vi "main_host.vi"() -> ()   [LabVIEW 2020]
uses:
  Status Cluster STYP.ctl
  Snake/Snake.lvclass
  INIFile/INIScoreFile.lvclass
  Drawing Settings STYP.ctl
  Food/Food.lvclass
  <userlib>/JET Engineering/JET_QSM/Code/Private/JET_QSM_InvalidOption STYP.ctl
  Direction STYP.ctl
  <userlib>/JET Engineering/JET_QSM/Code/Private/JET_QSM - Add State [String API].vi
  <vilib>/numeric/Random Number (Range) U64.vi
  <vilib>/numeric/sub_Random U32.vi
  <vilib>/Utility/error.llb/Trim Whitespace.vi
  <vilib>/Utility/error.llb/Error Cluster From Error Code.vi
panel:
  out "HighScores":i32(listbox)
  out "Score":u32
  out "Recent states before Error (with tick counts) 2":string="0.167 sec ago: VI Initialize\n0.167 sec ago: Window Open\n0.110 sec ago: Control Update\n0.110 sec ago: Indicator Update\n0.000 sec ago: Error Handler\r\n"
  in  "Status":T1
  out "error out":errorcluster
  out "Play Area":picture
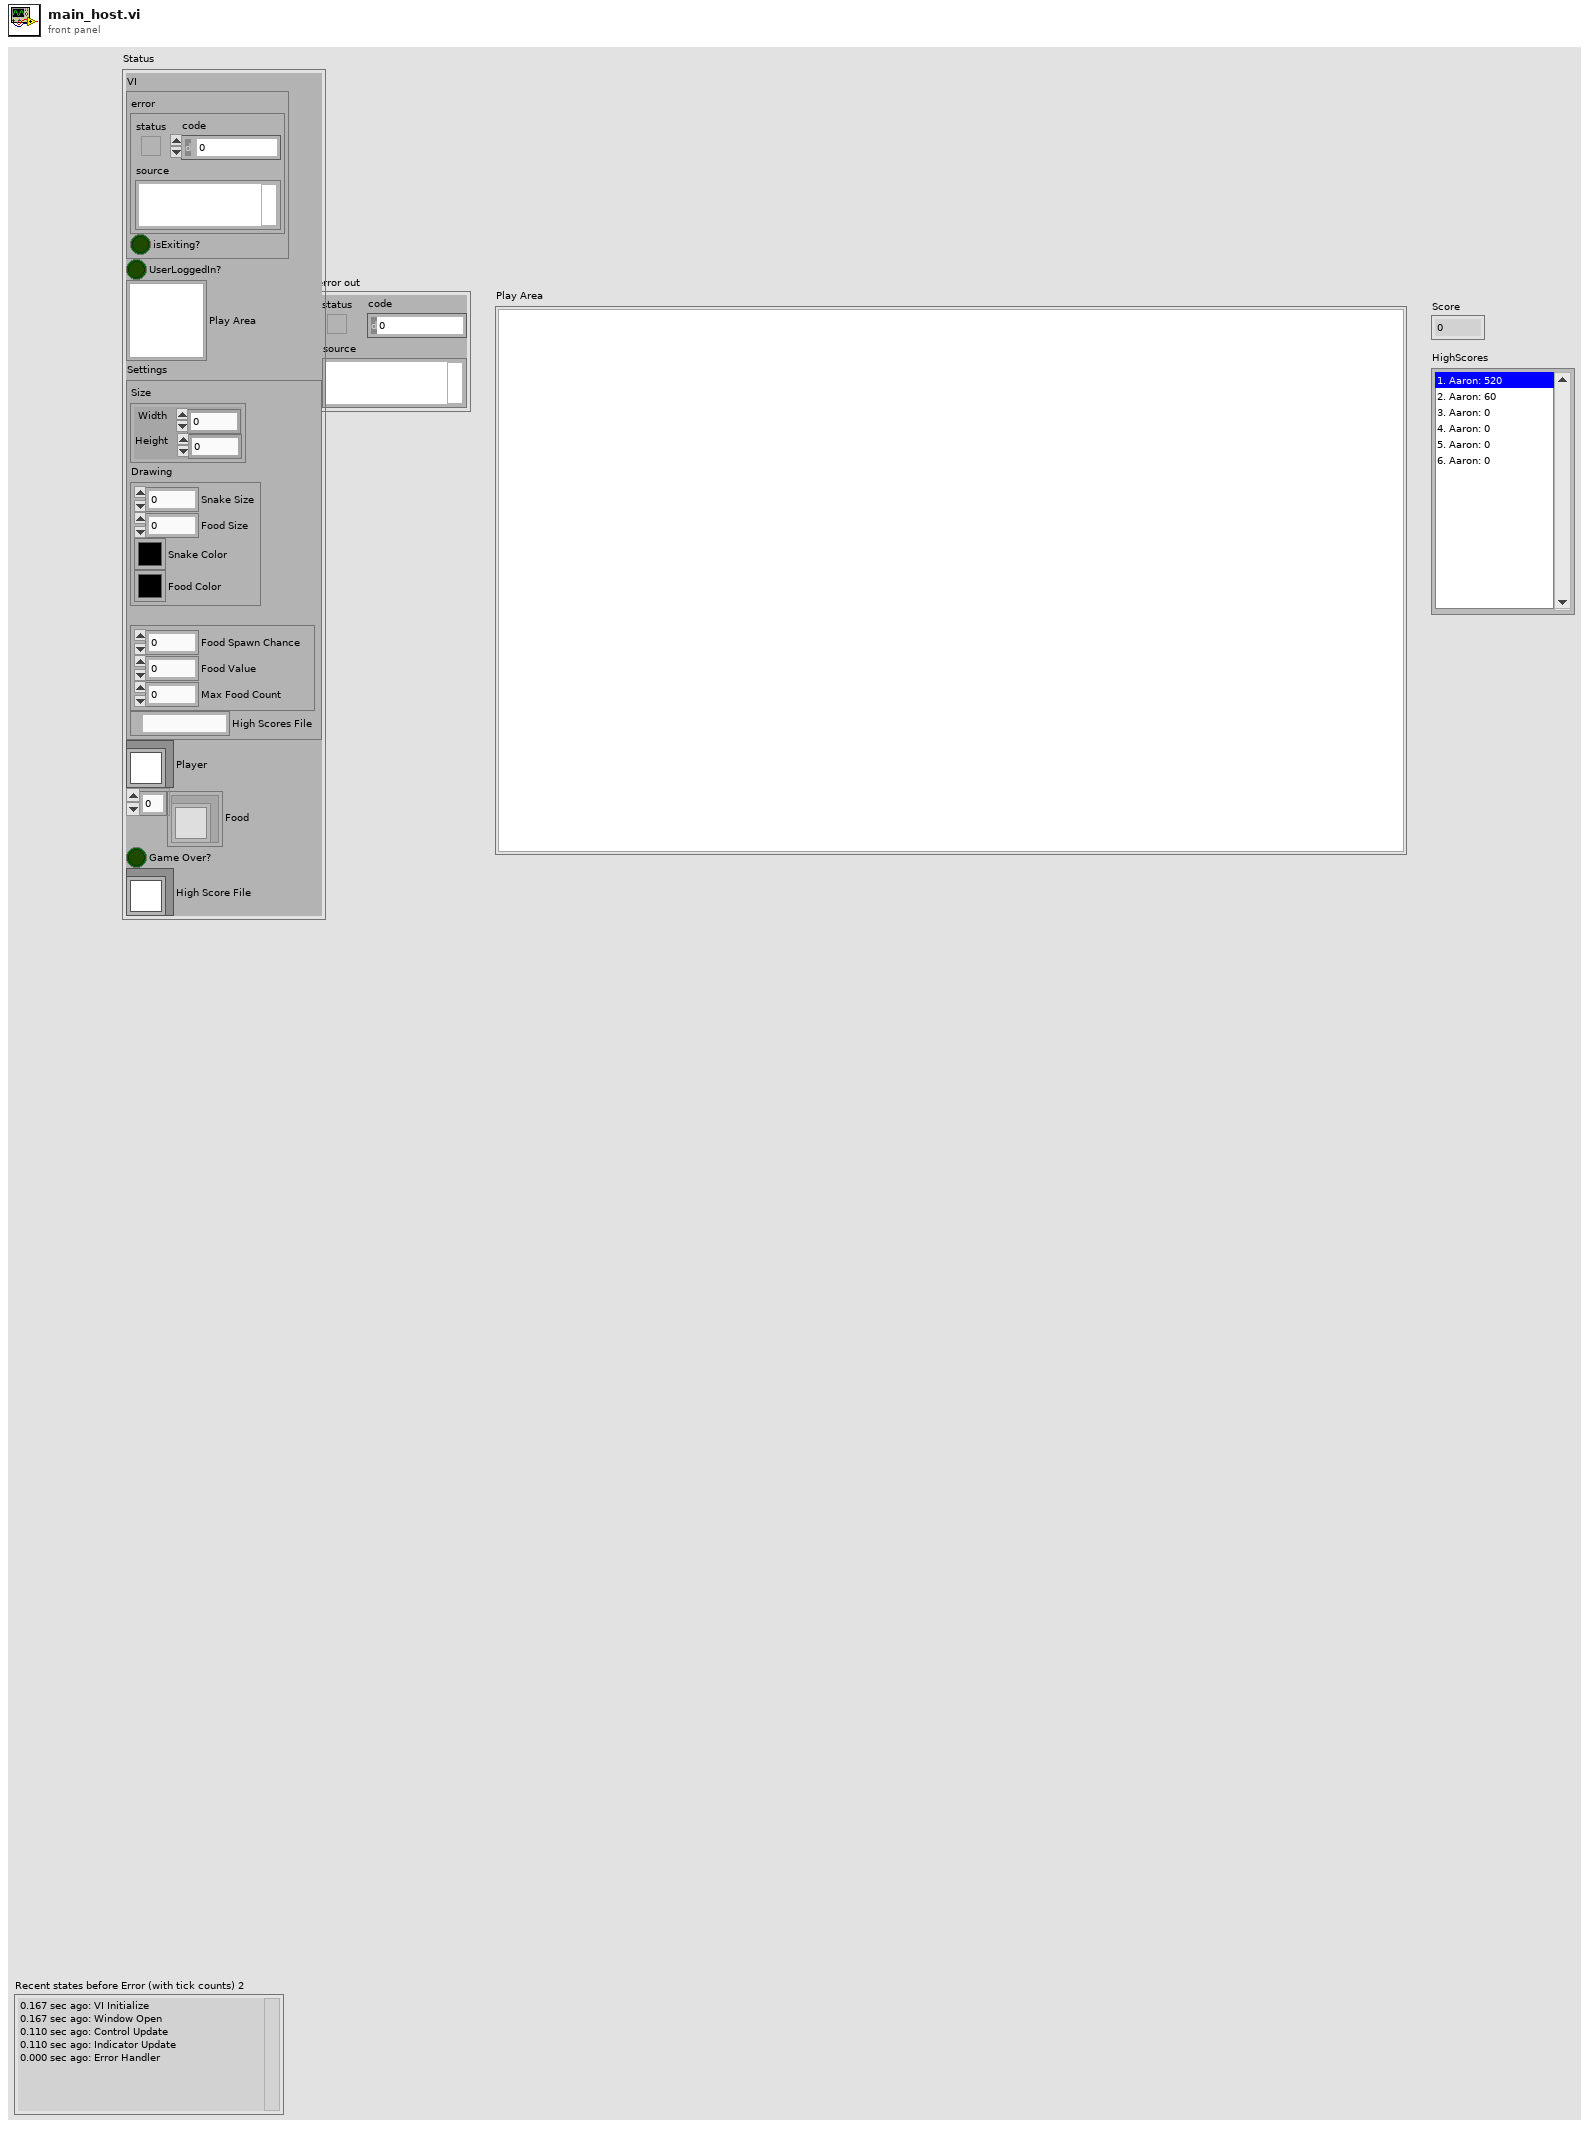
[diagram p1: front panel]
types:
  T1 = typedef "Status Cluster STYP.ctl" = cluster{"VI":cluster{"error":errorcluster, "isExiting?":bool}, "UserLoggedIn?":bool, "Play Area":picture, "Settings":cluster{"Size":cluster{"Width":u32, "Height":u32}, "Drawing":T2, "Food":cluster{"Food Spawn Chance":dbl, "Food Value":u32, "Max Food Count":i32}, "High Scores File":path}, "Player":refnum<class "Snake.lvclass">, "Food":refnum<class "Food.lvclass">[], "Game Over?":bool, "High Score File":refnum<class "INIScoreFile.lvclass">}
  T2 = typedef "Drawing Settings STYP.ctl" = cluster{"Snake Size":u32, "Food Size":u32, "Snake Color":u32, "Food Color":u32}
  T3 = typedef "JET_QSM_InvalidOption STYP.ctl" = enum16{"Ignore", "Dialog", "Error"}
  T4 = typedef "JET_QSM_Refnum STYP.ctl" = cluster{"state":cluster{"queue":refnum<queue>, "idle":string, "error":string, "STOP":string}, "debug":cluster{"enabled?":bool, "queue":refnum<queue>}, "Invalid.option":T3, "QSM.Name":string}
  T5 = enum32{"invalid app kind", "Development System", "Run Time System", "Student Edition", "Embedded LabVIEW", "Evaluation", "Custom"}
  T6 = typedef "Direction STYP.ctl" = enum16{"Up", "Down", "Left", "Right"}
  T7 = typedef "LVBoundsTypeDef.ctl" = cluster{"Width":u32, "Height":u32}
  T8 = typedef "eventvkey.ctl" = enum16{"ASCII", "Enter", "Return", "Shift", "Ctrl", "Alt", "Cmd", "Opt", "Caps", "NumLock", "Clear", "Break", "Up", "Down", "Left", "Right", "Insert", "Delete", "Home", "End", "PageUp", "PageDown", "Escape", "Help", "Pause", "ScrollLock", "F1", "F2", "F3", "F4", "F5", "F6", "F7", "F8", "F9", "F10", "F11", "F12", "F13", "F14", "F15", "F16", "F17", "F18", "F19", "F20", "F21", "F22", "F23", "F24", "Play", "VolumeUp", "VolumeDown", "Mute", "Two Byte Char"}
  T9 = typedef "JET_QSM_Element STYP.ctl" = cluster{"state":string, "data":variant, "comment":string}
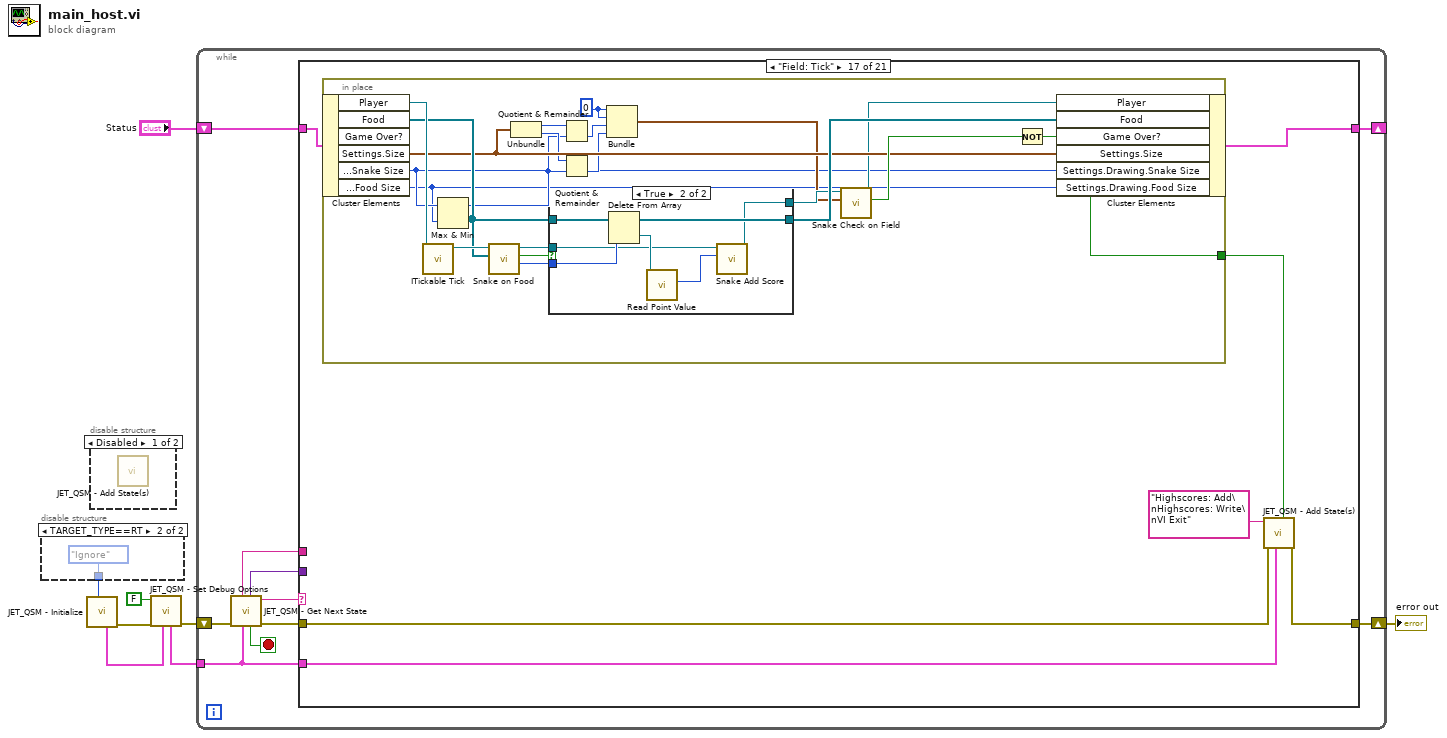
[diagram p0: block diagram]
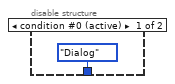
[diagram p2: hidden frame]
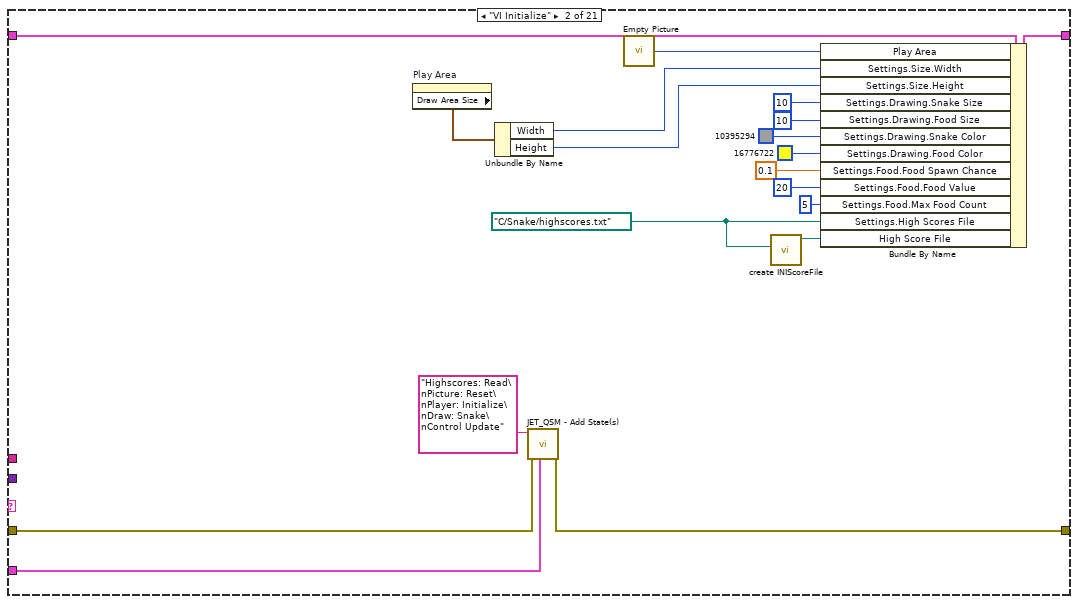
[diagram p5: hidden frame]
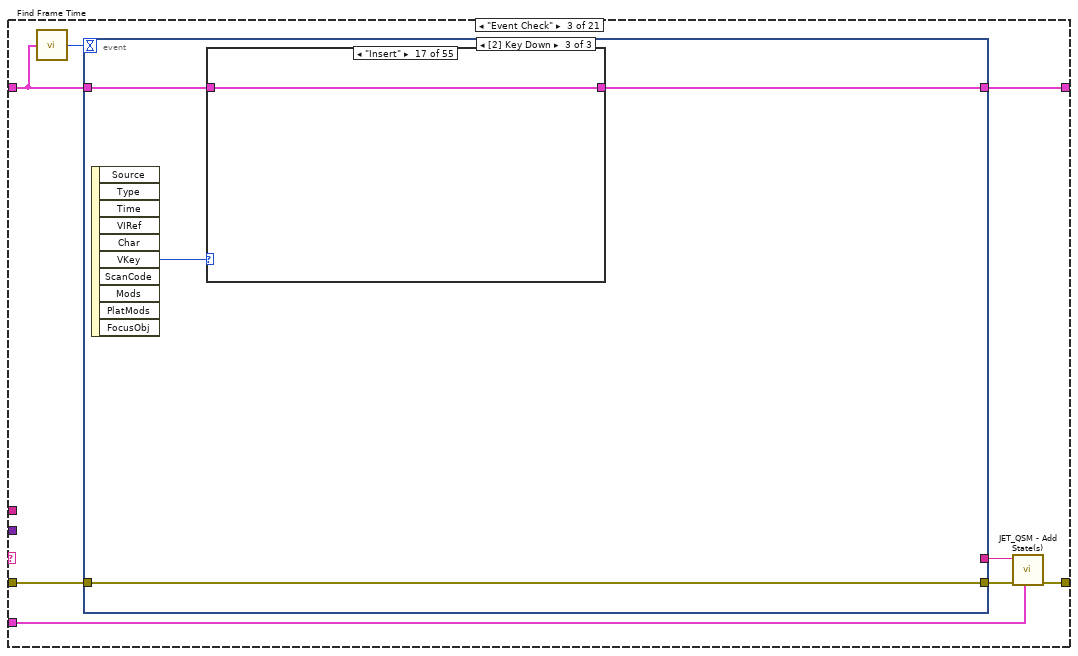
[diagram p6: hidden frame]
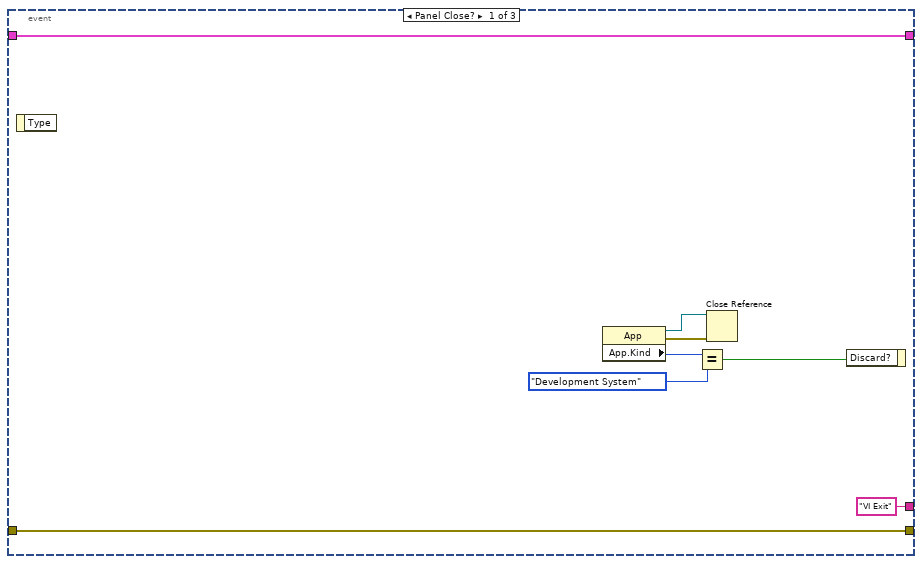
[diagram p7: hidden frame]
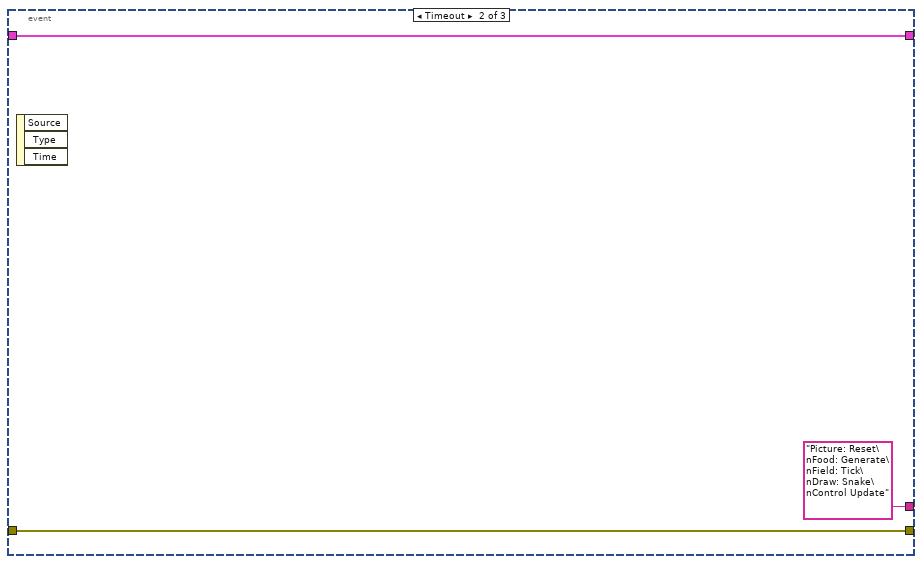
[diagram p8: hidden frame]
diagram:
  n1 = disable-structure shown="TARGET_TYPE==RT" {
    disable-tunnel: [JET_QSM_InvalidOption_STYP."Dialog" ("invalid state action (Dialog)") JET_QSM_InvalidOption_STYP."Ignore" ("invalid state action (Dialog)")] -> w8
    frame condition #0 (active) {
    }
    frame condition #1 {
    }
  }
  n2 = call <userlib>:"JET_QSM - Initialize.vi"("invalid state action (Dialog)"=w8) -> ("error out"=w1:errorcluster, "Jet_QSM refnum"=w4:T4)  [unwired: 9 in]
  n3 = disable-structure shown="Disabled" {
    frame Disabled {
      n4 = call-poly <userlib>:"JET_QSM - Add State(s).vi"() -> ()  [unwired: 11 in, 1 out]
    }
    frame Enabled {
    }
  }
  n5 = call <userlib>:"JET_QSM - Set Debug Options.vi"("Jet_QSM refnum"=w4, "error in (no error)"=w1, "debug.enabled? (F)"=FALSE) -> ("error out"=w2:errorcluster, "Jet_QSM ref"=w3:T4)  [unwired: 7 in]
  n6 = while {
    tunnel: w3 -> [w16]
    shift-right: [w14] -> _
    shift-left: "Status" -> [w15]
    shift-right: [w13] -> w7
    shift-left: w2 -> [w20]
    stop <- w17 stop-if-true
    n7 = call <userlib>:"JET_QSM - Get Next State.vi"("Jet_QSM refnum"=w16, "error in (no error)"=w20) -> ("error out"=w19:errorcluster, "state"=w18:string, "Stop Loop?"=w17:bool, "state data"=w12:variant, "state comment"=w11:string)  [unwired: 5 in]
    n8 = case shown="\"Field: Tick\"" w18 {
      selector: w18 -> [_ _ _ _ _ _ w176 _ _ _ _ _ _ _ _ _ _ _ _ _ _]
      tunnel: w19 -> [w21 w35 w49 w137 w168 _ w177 w179 w181 w183 w185 w197 w210 w225 w243 w254 w277 w312 w327 w330 w340]
      tunnel: w16 -> [_ w34 w48 w142 w166 _ w175 _ _ _ _ _ _ _ _ _ w276 _ _ w331 _]
      tunnel: w15 -> [w22 w41 w43 w138 w164 w172 w178 w180 w182 w184 w188 w200 w211 w226 w240 w252 w280 w313 w328 w333 w339]
      tunnel: [w22 w26 w44 w136 w164 w172 w178 w180 w182 w184 w187 w199 w209 w224 w242 w253 w279 w311 w328 w333 w339] -> w14
      tunnel: [w21 w36 w46 w143 w168 w173 w174 w179 w181 w183 w186 w198 w210 w225 w243 w254 w278 w312 w327 w329 w340] -> w13
      tunnel: w12 -> [_ _ _ _ _ _ _ _ _ _ _ _ _ _ _ _ _ _ _ _ _]
      tunnel: w11 -> [_ _ _ _ _ _ _ _ _ _ _ _ _ _ _ _ _ _ _ _ _]
      frame "------ Standard States ------" {
        # "Standard States are required states for a JET_QSM State Machine\n\nTheir names may be changed; use the Initialize function to specify the new names"
        # "This is a section header; the state is never expected to execute"
      }
      frame "VI Initialize" {
        w23 = path "C:/Snake/highscores.txt" ("Settings.High Scores File")
        n9 = property on="Play Area" class="Pict"() -> ("Draw Area Size"=w39:T7)  [unwired: 2 in, 2 out]
        n10 = Unbundle By Name(w39) -> ("Width"=w38:u32, "Height"=w37:u32)
        n11 = call-poly <userlib>:"JET_QSM - Add State(s).vi"("Jet_QSM refnum"=w34, "error in (no error)"=w35, "state(s)"="Highscores: Read\nPicture: Reset\nPlayer: Initialize\nDraw: Snake\nControl Update") -> ("error out"=w36:errorcluster)  [unwired: 8 in]
        n12 = call "Empty Picture"() -> ("empty picture"=w40:picture)
        n13 = call "create INIScoreFile.vi"("Path"=w23) -> ("INIScoreFile out"=w24:refnum<class "INIScoreFile.lvclass">)  [unwired: 9 in, 1 out]
        n14 = Bundle By Name(cluster=w41, "Play Area"=w40, "Settings.Size.Width"=w38, "Settings.Size.Height"=w37, "Settings.Drawing.Snake Size"=u32 10, "Settings.Drawing.Food Size"=u32 10, "Settings.Drawing.Snake Color"=u32 10395294, "Settings.Drawing.Food Color"=u32 16776722, "Settings.Food.Food Spawn Chance"=0.1 ("Settings.Food Spawn Chance"), "Settings.Food.Food Value"=u32 20 ("Settings.Food Value"), "Settings.Food.Max Food Count"=5, "Settings.High Scores File"=w23, "High Score File"=w24) -> (w26:T1)
      }
      frame "Event Check" {
        n15 = call "Find Frame Time.vi"("Status"=w43) -> ("Frame Time (ms)"=w42:i32)
        n16 = event shown="[2] Key Down" {
          selector: _ -> [_ _ _]
          dyn-events: _ -> [_ _ _]
          timeout: w42 -> [_ _ _]
          tunnel: w49 -> [w51 w60 w61]
          tunnel: ["VI Exit" ("state(s)") "Picture: Reset\nFood: Generate\nField: Tick\nDraw: Snake\nControl Update" ("state(s)") _] -> w47
          tunnel: [w51 w60 w61] -> w45
          tunnel: w43 -> [w50 w58 w63]
          tunnel: [w50 w58 w62] -> w44
          event Panel Close? {
            n17 = event-data() -> ()  [unwired: 1 in, 1 out]
            n18 = property class="App"() -> (reference out=w53:refnum<vi>, error out=w54:errorcluster, "App.Kind"=w57:T5)  [unwired: 2 in]
            n19 = Equal?(x=w57, y=T5."Development System") -> (x = y?=w55:bool)
            n20 = Close Reference(reference=w53, error in (no error)=w54) -> ()  [unwired: 1 out]
            n21 = event-data("Discard?"=w55) -> ()  [unwired: 1 in, 1 out]
          }
          event Timeout {
            n22 = event-data() -> ()  [unwired: 1 in, 3 out]
          }
          event Key Down {
            n23 = event-data() -> ("VKey"=w64:T8)  [unwired: 1 in, 9 out]
            n24 = case shown="\"Insert\"" w64 {
              tunnel: w63 -> [w65 w66 w67 w68 w69 w70 w71 w72 w73 w74 w75 w76 w78 w83 w88 w93 w97 w98 w99 w100 w101 w102 w103 w104 w105 w106 w107 w108 w109 w110 w111 w112 w113 w114 w115 w116 w117 w118 w119 w120 w121 w122 w123 w124 w125 w126 w127 w128 w129 w130 w131 w132 w133 w134 w135]
              tunnel: [w65 w66 w67 w68 w69 w70 w71 w72 w73 w74 w75 w76 w77 w82 w87 w92 w97 w98 w99 w100 w101 w102 w103 w104 w105 w106 w107 w108 w109 w110 w111 w112 w113 w114 w115 w116 w117 w118 w119 w120 w121 w122 w123 w124 w125 w126 w127 w128 w129 w130 w131 w132 w133 w134 w135] -> w62
              frame "ASCII", Default {
              }
              frame "Enter" {
              }
              frame "Return" {
              }
              frame "Shift" {
              }
              frame "Ctrl" {
              }
              frame "Alt" {
              }
              frame "Cmd" {
              }
              frame "Opt" {
              }
              frame "Caps" {
              }
              frame "NumLock" {
              }
              frame "Clear" {
              }
              frame "Break" {
              }
              frame "Up" {
                n25 = in-place {
                  n26 = in-place-cluster #1(w78) -> ("Player"=w81:refnum<class "Snake.lvclass">)
                  n27 = call-dynamic "Snake Change Direction.vi"("Direction"=Direction_STYP."Up", "Snake in"=w81) -> ("Snake out"=w80:refnum<class "Snake.lvclass">)  [unwired: 8 in, 1 out]
                  n28 = in-place-cluster #1("Player"=w80) -> (w77:T1)
                }
              }
              frame "Down" {
                n29 = in-place {
                  n30 = in-place-cluster #2(w83) -> ("Player"=w86:refnum<class "Snake.lvclass">)
                  n31 = call-dynamic "Snake Change Direction.vi"("Direction"=Direction_STYP."Down", "Snake in"=w86) -> ("Snake out"=w85:refnum<class "Snake.lvclass">)  [unwired: 8 in, 1 out]
                  n32 = in-place-cluster #2("Player"=w85) -> (w82:T1)
                }
              }
              frame "Left" {
                n33 = in-place {
                  n34 = in-place-cluster #3(w88) -> ("Player"=w91:refnum<class "Snake.lvclass">)
                  n35 = call-dynamic "Snake Change Direction.vi"("Direction"=Direction_STYP."Left", "Snake in"=w91) -> ("Snake out"=w90:refnum<class "Snake.lvclass">)  [unwired: 8 in, 1 out]
                  n36 = in-place-cluster #3("Player"=w90) -> (w87:T1)
                }
              }
              frame "Right" {
                n37 = in-place {
                  n38 = in-place-cluster #4(w93) -> ("Player"=w96:refnum<class "Snake.lvclass">)
                  n39 = call-dynamic "Snake Change Direction.vi"("Direction"=Direction_STYP."Right", "Snake in"=w96) -> ("Snake out"=w95:refnum<class "Snake.lvclass">)  [unwired: 8 in, 1 out]
                  n40 = in-place-cluster #4("Player"=w95) -> (w92:T1)
                }
              }
              frame "Insert" {
              }
              frame "Delete" {
              }
              frame "Home" {
              }
              frame "End" {
              }
              frame "PageUp" {
              }
              frame "PageDown" {
              }
              frame "Escape" {
              }
              frame "Help" {
              }
              frame "Pause" {
              }
              frame "ScrollLock" {
              }
              frame "F1" {
              }
              frame "F2" {
              }
              frame "F3" {
              }
              frame "F4" {
              }
              frame "F5" {
              }
              frame "F6" {
              }
              frame "F7" {
              }
              frame "F8" {
              }
              frame "F9" {
              }
              frame "F10" {
              }
              frame "F11" {
              }
              frame "F12" {
              }
              frame "F13" {
              }
              frame "F14" {
              }
              frame "F15" {
              }
              frame "F16" {
              }
              frame "F17" {
              }
              frame "F18" {
              }
              frame "F19" {
              }
              frame "F20" {
              }
              frame "F21" {
              }
              frame "F22" {
              }
              frame "F23" {
              }
              frame "F24" {
              }
              frame "Play" {
              }
              frame "VolumeUp" {
              }
              frame "VolumeDown" {
              }
              frame "Mute" {
              }
              frame "Two Byte Char" {
              }
            }
          }
        }
        n41 = call-poly <userlib>:"JET_QSM - Add State(s).vi"("Jet_QSM refnum"=w48, "error in (no error)"=w45, "state(s)"=w47) -> ("error out"=w46:errorcluster)  [unwired: 8 in]
      }
      frame "Error Handler" {
        # "Add specific error exception handlers here"
        n42 = Get Date/Time In Seconds() -> (seconds since 1Jan1904=w146:timestamp)
        n43 = call <userlib>:"JET_QSM - Flush Debug Queue.vi"("Jet_QSM refnum"=w142) -> ("QSM Elements"=w144:T9[], "Timestamps"=w145:timestamp[])  [unwired: 8 in, 1 out]
        n44 = Bundle By Name(cluster=w138, "VI.error"=w137) -> (w136:T1)
        n45 = Unbundle By Name(w137) -> ("code"=w139:i32)
        n46 = for {
          tunnel: w144 -> [w158] mode=indexing
          tunnel: [w156] -> w148 mode=indexing
          tunnel: w146 -> [w153]
          tunnel: w145 -> [w154] mode=indexing
          n47 = Subtract(x=w153, y=w154) -> (x-y=w152:dbl)
          n48 = To Double Precision Float(number=w152) -> (double precision float=w151:dbl)
          n49 = Unbundle By Name(w158) -> ("state"=w157:string)
          n50 = Format Into String(format string="%.03f sec ago: %s", w151, w157) -> (resulting string=w156:string)  [unwired: 2 in, 1 out]
        }
        n51 = case shown="Default" w139 {
          selector: w139 -> [w160]
          tunnel: [w161] -> w140
          tunnel: w137 -> [w159]
          frame Default {
            w161 = TRUE  # Exit?
            n52 = disable-structure shown="Default" {
              disable-tunnel: w160 -> [w163 _]
              disable-tunnel: w159 -> [w162 _]
              frame condition #0 (active) {
                n53 = call <vilib>:"Simple Error Handler.vi"("error code (no error:0)"=w163, "error in (no error)"=w162) -> ()  [unwired: 3 in, 5 out]
              }
              frame condition #1 {
              }
            }
          }
        }
        n54 = Array To Spreadsheet String(delimiter (Tab)="\n", array=w148, 3:"%s" ("format string")) -> (spreadsheet string=→"Recent states before Error (with tick counts) 2":string)
        n55 = call-poly <userlib>:"JET_QSM - Add State(s).vi"("act? (T)"=w140, "Jet_QSM refnum"=w142, "state(s)"="VI Exit") -> ("error out"=w143:errorcluster)  [unwired: 8 in]
      }
      frame "VI Exit" {
        n56 = flat-sequence {
          tunnel: w168 -> [w171]
          tunnel: [w170] -> w167
          tunnel: w166 -> [w169]
          tunnel: [w169] -> w165
          frame #0 {
            n57 = call <userlib>:"JET_QSM - Flush.vi"("Jet_QSM ref"=w169, "error in (no error)"=w171) -> ("error out"=w170:errorcluster)  [unwired: 8 in, 1 out]
          }
        }
        n58 = call <userlib>:"JET_QSM - Add STOP.vi"("Jet_QSM refnum"=w165, "error in (no error)"=w167) -> ()  [unwired: 9 in, 1 out]
      }
      frame "VI STOP" {
        # "Pass out any error that was cached"
        # "This State is the STOP State.\nIt ALWAYS is the last state to execute."
        n59 = Unbundle By Name(w172) -> ("VI.error"=w173:errorcluster)
      }
      frame "INVALID STATE", Default {
        # "This is the state that handles a state name that is INVALID (there is no state for it in the state machine)"
        n60 = call <userlib>:"JET_QSM - INVALID State.vi"("Jet_QSM refnum"=w175, "error in (no error)"=w177, "state"=w176) -> ("error out"=w174:errorcluster)  [unwired: 8 in]
      }
      frame "------ Menu Commands ------" {
        # "This is a section header; the state is never expected to execute"
      }
      frame "------ Events  ------" {
        # "This is a section header; the state is never expected to execute"
      }
      frame "------ Actions  ------" {
        # "This is a section header; the state is never expected to execute"
      }
      frame "Highscores: Read" {
        n61 = in-place {
          in-place-border: w185 -> [w193]
          in-place-border: [w190] -> w186
          n62 = in-place-cluster #5(w188) -> ("High Score File"=w196:refnum<class "INIScoreFile.lvclass">)
          n63 = call-dynamic "IFile Open.vi"("error in (no error)"=w193, "INIScoreFile in"=w196) -> ("error out"=w194:errorcluster, "INIScoreFile out"=w195:refnum<class "INIScoreFile.lvclass">)  [unwired: 8 in]
          n64 = call-dynamic "IFile Read.vi"("error in (no error)"=w194, "INIScoreFile in"=w195) -> ("error out"=w191:errorcluster, "INIScoreFile out"=w192:refnum<class "INIScoreFile.lvclass">)  [unwired: 8 in]
          n65 = call-dynamic "IFile Close.vi"("error in (no error)"=w191, "INIScoreFile in"=w192) -> ("error out"=w190:errorcluster, "INIScoreFile out"=w189:refnum<class "INIScoreFile.lvclass">)  [unwired: 8 in]
          n66 = in-place-cluster #5("High Score File"=w189) -> (w187:T1)
        }
      }
      frame "Highscores: Write" {
        n67 = in-place {
          in-place-border: w197 -> [w205]
          in-place-border: [w202] -> w198
          n68 = in-place-cluster #6(w200) -> ("High Score File"=w208:refnum<class "INIScoreFile.lvclass">)
          n69 = call-dynamic "IFile Open.vi"("error in (no error)"=w205, "INIScoreFile in"=w208) -> ("error out"=w206:errorcluster, "INIScoreFile out"=w207:refnum<class "INIScoreFile.lvclass">)  [unwired: 8 in]
          n70 = call-dynamic "IFile Write.vi"("error in (no error)"=w206, "INIScoreFile in"=w207) -> ("error out"=w203:errorcluster, "INIScoreFile out"=w204:refnum<class "INIScoreFile.lvclass">)  [unwired: 8 in]
          n71 = call-dynamic "IFile Close.vi"("error in (no error)"=w203, "INIScoreFile in"=w204) -> ("error out"=w202:errorcluster, "INIScoreFile out"=w201:refnum<class "INIScoreFile.lvclass">)  [unwired: 8 in]
          n72 = in-place-cluster #6("High Score File"=w201) -> (w199:T1)
        }
      }
      frame "Highscores: Add" {
        n73 = in-place {
          n74 = in-place-cluster #7(w211) -> ("High Score File"=w217:refnum<class "INIScoreFile.lvclass">, "Player"=w216:refnum<class "Snake.lvclass">)
          n75 = call-dynamic "Read Score.vi"("Snake in"=w216) -> ("Score"=w213:u32)  [unwired: 8 in, 2 out]
          n76 = call-dynamic "INIScoreFile Check Score.vi"("Score"=w213, "INIScoreFile in"=w217) -> ("Is High?"=w215:bool, "INIScoreFile out"=w214:refnum<class "INIScoreFile.lvclass">)  [unwired: 7 in, 1 out]
          n77 = case shown="False" w215 {
            tunnel: w214 -> [w218 w222]
            tunnel: w213 -> [_ w220]
            tunnel: [w218 w219] -> w212
            frame False {
            }
            frame True {
              n78 = call "HighScore Name Entry"() -> ("Name"=w221:string)  [unwired: 17 in, 2 out]
              n79 = call-dynamic "INIScoreFile Add Score.vi"("Score"=w220, "Name"=w221, "INIScoreFile in"=w222) -> ("INIScoreFile out"=w219:refnum<class "INIScoreFile.lvclass">)  [unwired: 7 in, 1 out]
            }
          }
          n80 = in-place-cluster #7("High Score File"=w212, "Player"=w216) -> (w209:T1)
        }
      }
      frame "Picture: Reset" {
        n81 = Bundle By Name(cluster=w226, "Play Area"=picture data[5B]) -> (w224:T1)
      }
      frame "Player: Initialize" {
        w227 = 10
        n82 = Unbundle By Name(w240) -> ("Settings.Size.Width"=w237:u32, "Settings.Size.Height"=w236:u32, "Settings.Drawing.Snake Size"=w238:u32, "Settings.Drawing.Food Size"=w239:u32)
        n83 = Max & Min(x=w238, y=w239) -> (max(x,y)=w235:u32)  [unwired: 1 out]
        n84 = Quotient & Remainder(x=w236, y=w235) -> (floor(x/y)=w233:u32)  [unwired: 1 out]
        n85 = Quotient & Remainder(x=w237, y=w235) -> (floor(x/y)=w234:u32)  [unwired: 1 out]
        n86 = Decrement(x=w233) -> (x-1=w228:u32)
        n87 = Decrement(x=w234) -> (x-1=w229:u32)
        n88 = call-poly <vilib>:"Random Number (Range).vi"("lower bound (0)"=w227, "upper bound (100)"=w229) -> ("number"=w232:u64)  [unwired: 9 in]
        n89 = call-poly <vilib>:"Random Number (Range).vi"("lower bound (0)"=w227, "upper bound (100)"=w228) -> ("number"=w231:u64)  [unwired: 9 in]
        n90 = Bundle("number"=w232, "number"=w231) -> (w230:cluster{"number":u64, "number":u64})  [unwired: 1 in]
        n91 = call "create Snake.vi"("Starting Point"=w230) -> ("Snake out"=w241:refnum<class "Snake.lvclass">)  [unwired: 9 in, 1 out]
        n92 = Bundle By Name(cluster=w240, "Player"=w241) -> (w242:T1)
      }
      frame "Food: Generate" {
        n93 = Unbundle By Name(w252) -> ("Settings.Food.Food Spawn Chance"=w250:dbl, "Settings.Food.Max Food Count"=w246:i32, "Food"=w248:refnum<class "Food.lvclass">[])
        n94 = Array Size(array=w248) -> (size(s)=w247:i32)
        n95 = Random Number (0-1)() -> (number: 0 to 1=w251:dbl)
        n96 = Less?(x=w247, y=w246) -> (x < y?=w244:bool)
        n97 = Less Or Equal?(x=w251, y=w250) -> (x <= y?=w249:bool)
        n98 = And(x=w249, y=w244) -> (x .and. y?=w245:bool)
        n99 = case shown="True" w245 {
          tunnel: [w255 w273] -> w253
          tunnel: w252 -> [w255 w258]
          frame False {
          }
          frame True {
            n100 = Unbundle By Name(w258) -> ("Food"=w263:refnum<class "Food.lvclass">[], "Settings.Size.Width"=w270:u32, "Settings.Size.Height"=w269:u32, "Settings.Drawing.Snake Size"=w271:u32, "Settings.Drawing.Food Size"=w272:u32, "Settings.Food.Food Value"=w259:u32)
            n101 = Max & Min(x=w271, y=w272) -> (max(x,y)=w268:u32)  [unwired: 1 out]
            n102 = Quotient & Remainder(x=w269, y=w268) -> (floor(x/y)=w266:u32)  [unwired: 1 out]
            n103 = Quotient & Remainder(x=w270, y=w268) -> (floor(x/y)=w267:u32)  [unwired: 1 out]
            n104 = Decrement(x=w266) -> (x-1=w256:u32)
            n105 = Decrement(x=w267) -> (x-1=w257:u32)
            n106 = call-poly <vilib>:"Random Number (Range).vi"("upper bound (100)"=w256) -> ("number"=w264:u64)  [unwired: 10 in]
            n107 = call-poly <vilib>:"Random Number (Range).vi"("upper bound (100)"=w257) -> ("number"=w265:u64)  [unwired: 10 in]
            n108 = Bundle("number"=w265, "number"=w264) -> (w260:cluster{"number":u64, "number":u64})  [unwired: 1 in]
            n109 = call "create Food.vi"("Point Value"=w259, "Starting Point"=w260) -> ("Food out"=w261:refnum<class "Food.lvclass">)  [unwired: 8 in, 1 out]
            n110 = Build Array (concatenate)(w263, w261) -> (w262:refnum<class "Food.lvclass">[])
            n111 = Bundle By Name(cluster=w258, "Food"=w262) -> (w273:T1)
          }
        }
      }
      frame "Field: Tick" {
        n112 = in-place {
          in-place-border: [w288] -> w274
          w291 = u32 0
          n113 = in-place-cluster #8(w280) -> ("Player"=w301:refnum<class "Snake.lvclass">, "Food"=w296:refnum<class "Food.lvclass">[], "Settings.Size"=w292:cluster{"Width":u32, "Height":u32}, "Settings.Drawing.Snake Size"=w282:u32, "Settings.Drawing.Food Size"=w281:u32)  [unwired: 1 out]
          n114 = call-dynamic "ITickable Tick.vi"("Snake in"=w301) -> ("Snake out"=w300:refnum<class "Snake.lvclass">)  [unwired: 9 in, 1 out]
          n115 = Max & Min(x=w282, y=w281) -> (max(x,y)=w283:u32)  [unwired: 1 out]
          n116 = call-dynamic "Snake on Food.vi"("Food Locations"=w296, "Snake in"=w300) -> ("Food Index"=w298:i32, "On Food?"=w299:bool, "Snake out"=w297:refnum<class "Snake.lvclass">)  [unwired: 6 in, 1 out]
          n117 = Unbundle(w292) -> ("Width"=w287:u32, "Height"=w284:u32)
          n118 = case shown="True" w299 {
            tunnel: w298 -> [_ w309]
            tunnel: w297 -> [w302 w306]
            tunnel: w296 -> [w303 w310]
            tunnel: [w303 w307] -> w295
            tunnel: [w302 w304] -> w294
            frame False {
            }
            frame True {
              n119 = Delete From Array(array=w310, index=w309) -> (deleted portion=w308:refnum<class "Food.lvclass">, array with subset deleted=w307:refnum<class "Food.lvclass">[])  [unwired: 1 in]
              n120 = call-dynamic "Read Point Value.vi"("Food in"=w308) -> ("Point Value"=w305:u32)  [unwired: 8 in, 2 out]
              n121 = call-dynamic "Snake Add Score.vi"("Amount"=w305, "Snake in"=w306) -> ("Snake out"=w304:refnum<class "Snake.lvclass">)  [unwired: 8 in, 1 out]
            }
          }
          n122 = Quotient & Remainder(x=w287, y=w283) -> (floor(x/y)=w286:u32)  [unwired: 1 out]
          n123 = Quotient & Remainder(x=w284, y=w283) -> (floor(x/y)=w285:u32)  [unwired: 1 out]
          n124 = Bundle(w291, w291, w286, w285) -> (w290:cluster{u32, u32, u32, u32})  [unwired: 1 in]
          n125 = call-dynamic "Snake Check on Field.vi"("Bounds"=w290, "Snake in"=w294) -> ("On Field?"=w293:bool, "Snake out"=w289:refnum<class "Snake.lvclass">)  [unwired: 7 in, 1 out]
          n126 = Not(x=w293) -> (.not. x?=w288:bool)
          n127 = in-place-cluster #8("Player"=w289, "Food"=w295, "Game Over?"=w288, "Settings.Size"=w292, "Settings.Drawing.Snake Size"=w282, "Settings.Drawing.Food Size"=w281) -> (w279:T1)
        }
        n128 = call-poly <userlib>:"JET_QSM - Add State(s).vi"("act? (T)"=w274, "Jet_QSM refnum"=w276, "error in (no error)"=w277, "state(s)"="Highscores: Add\nHighscores: Write\nVI Exit") -> ("error out"=w278:errorcluster)  [unwired: 7 in]
      }
      frame "Draw: Snake" {
        n129 = in-place {
          n130 = in-place-cluster #9(w313) -> ("Play Area"=w320:picture, "Settings.Drawing"=w316:T2, "Player"=w321:refnum<class "Snake.lvclass">, "Food"=w318:refnum<class "Food.lvclass">[])
          n131 = call-dynamic "IDrawable Draw.vi"("Drawing Settings"=w316, "2D Picture"=w320, "Snake in"=w321) -> ("2D Picture out"=w317:picture, "Snake out"=w319:refnum<class "Snake.lvclass">)  [unwired: 6 in, 1 out]
          n132 = for {
            tunnel: w318 -> [w326] mode=indexing
            shift-right: [w323] -> w314
            shift-left: w317 -> [w324]
            tunnel: w316 -> [w325]
            tunnel: [w322] -> w315 mode=indexing
            n133 = call-dynamic "IDrawable Draw.vi"("Drawing Settings"=w325, "2D Picture"=w324, "Food in"=w326) -> ("2D Picture out"=w323:picture, "Food out"=w322:refnum<class "Food.lvclass">)  [unwired: 6 in, 1 out]
          }
          n134 = in-place-cluster #9("Play Area"=w314, "Settings.Drawing"=w316, "Player"=w319, "Food"=w315) -> (w311:T1)
        }
      }
      frame "------ Window and Panel Control ------" {
        # "This is a section header; the state is never expected to execute"
      }
      frame "Control Update" {
        # "Update all control properties here from the status cluster\n(Consolidate/reduce property nodes)"
        n135 = call-poly <userlib>:"JET_QSM - Add State(s).vi"("Jet_QSM refnum"=w331, "error in (no error)"=w330, "state(s)"="Indicator Update") -> ("error out"=w329:errorcluster)  [unwired: 8 in]
      }
      frame "Indicator Update" {
        # "Update all indicator values here from the status cluster\n(Eliminate Local Variables)"
        n136 = Unbundle By Name(w339) -> ("Play Area"=→"Play Area":picture, "Player"=w337:refnum<class "Snake.lvclass">, "High Score File"=w335:refnum<class "INIScoreFile.lvclass">)
        n137 = call-dynamic "Read Score.vi"("Snake in"=w337) -> ("Score"=→"Score":u32)  [unwired: 8 in, 2 out]
        n138 = call-dynamic "INIScoreFile Get Strings.vi"("INIScoreFile in"=w335) -> ("Lines"=w334:string[])  [unwired: 8 in, 2 out]
        n139 = property on="HighScores" class="LstBox (strict)"("Item Names"=w334) -> ()  [unwired: 2 in, 2 out]
      }
    }
  }
  "error out" <- w7
